vi "Find Child of Node With Children.vi"(8 "error in":errorcluster, 10 "Node":T2, 11 "Fast Tree in":refnum<class "Fast Tree.lvclass">) -> (0 "error out":errorcluster, 2 "Children":T1(array[cluster]), 3 "Fast Tree out":refnum<class "Fast Tree.lvclass">)   [LabVIEW 2019, in "Fast Tree.lvclass"]
uses:
  Fast Tree.lvclass
  Fast Tree.lvclass/Fast Tree.ctl
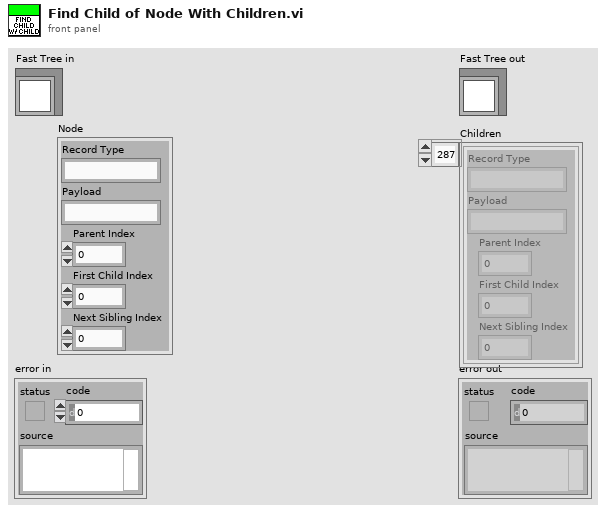
[diagram p1: front panel]
types:
  T1 = cluster{"Record Type":string, "Payload":string, "Parent Index":i32, "First Child Index":i32, "Next Sibling Index":i32}[]
  T2 = cluster{"Record Type":string, "Payload":string, "Parent Index":i32, "First Child Index":i32, "Next Sibling Index":i32}
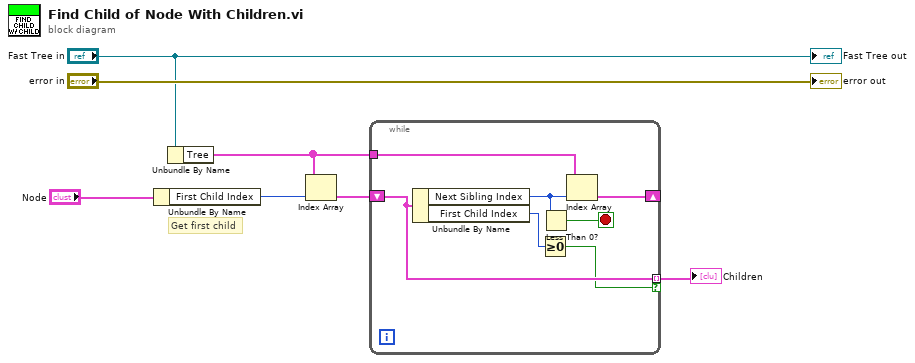
[diagram p0: block diagram]
diagram:
  # "Get first child"
  n1 = Unbundle By Name("Node") -> ("First Child Index"=w4:i32)
  n2 = Unbundle By Name("Fast Tree in") -> ("Tree"=w5:T1)
  n3 = Index Array(array=w5, index=w4) -> (element=w6:T2)
  n4 = while {
    tunnel: [w13] -> w1 mode=indexing if=w8
    tunnel: w5 -> [w12]
    shift-right: [w11] -> _
    shift-left: w6 -> [w13]
    stop <- w14 stop-if-true
    n5 = Unbundle By Name(w13) -> ("Next Sibling Index"=w10:i32, "First Child Index"=w9:i32)
    n6 = Greater Or Equal To 0?(x=w9) -> (x >= 0?=w8:bool)
    n7 = Less Than 0?(x=w10) -> (x < 0?=w14:bool)
    n8 = Index Array(array=w12, index=w10) -> (element=w11:T2)
  }
  "Children" <- w1
  "error out" <- "error in"
  "Fast Tree out" <- "Fast Tree in"
